vi "GT_Read IOPort.vi"(1 "I/O Port":i32) -> (0 "I/O Status":bool)   [LabVIEW 2014]
uses:
  VC6/gts.dll
panel:
  out "ArrayOut":bool[](array[boolean])
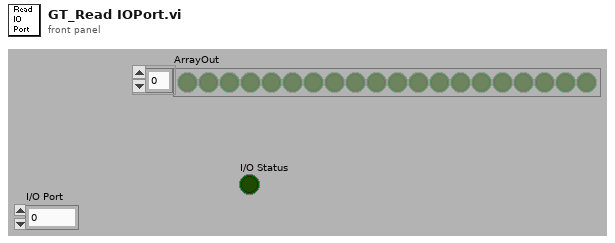
[diagram p1: front panel]
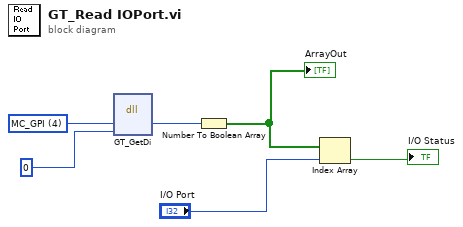
[diagram p0: block diagram]
diagram:
  w6 = u16 4 items=["MC_LIMIT_POSITIVE", "MC_LIMIT_NEGATIVE", "MC_ALARM", "MC_HOME", "MC_GPI", "MC_ARRIVE"]
  n1 = dll-call lib="PTH2Fabs DNewGTS AC-800LWin7版源程序-20170926gts85VC6gts.dll" fn="GT_GetDi"("diType"=w6, "pValue"=0) -> ("diType"=w4:i16)  [unwired: 5 in, 2 out]
  n2 = Number To Boolean Array(number=w4) -> (Boolean array=w3:bool[])
  "ArrayOut" <- w3
  n3 = Index Array(array=w3, index="I/O Port") -> (element=→"I/O Status":bool)
